vi "Arial Assist Ball Fetch.vi"() -> ()   [LabVIEW 2013]
uses:
  <vilib>/Rock Robotics/WPI/RobotDrive/WPI_RobotDriveMecanumDrive_Cartesian.vi
panel:
  in  "Vision?":bool
  in  "Far X":dbl
  in  "Far Less":dbl
  in  "Far Greater":dbl
  in  "Close Greater":dbl
  in  "Close Less":dbl
  in  "Close Threshold":dbl
  in  "Stopping Threshold":dbl
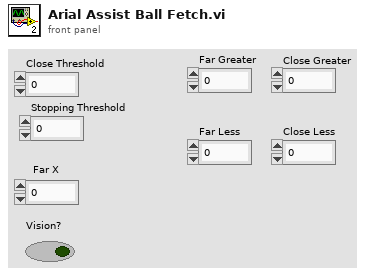
[diagram p1: front panel]
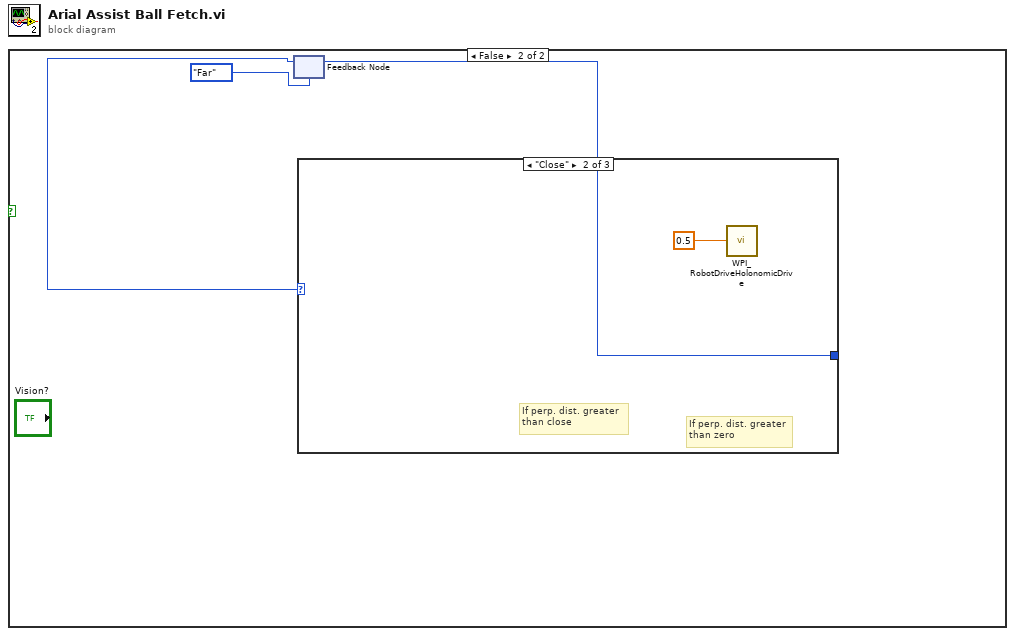
[diagram p0: block diagram]
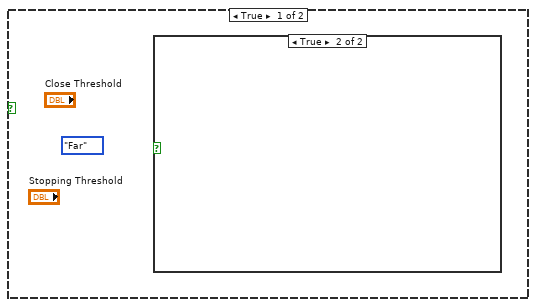
[diagram p2: hidden frame]
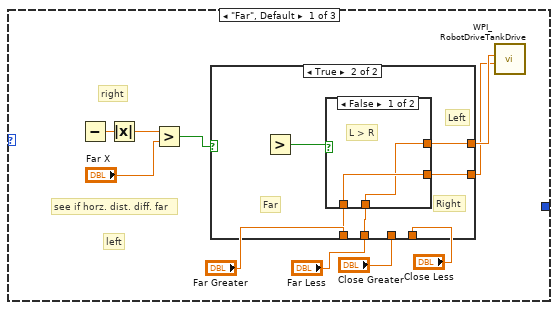
[diagram p4: hidden frame]
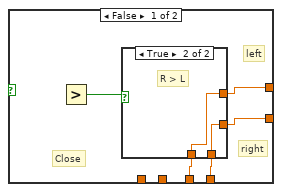
[diagram p5: hidden frame]
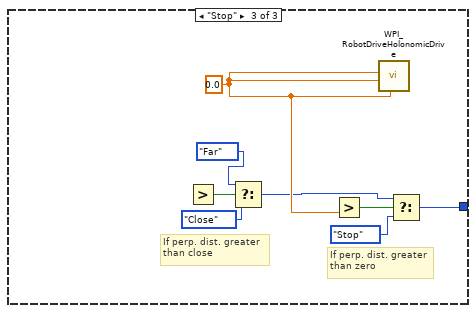
[diagram p8: hidden frame]
diagram:
  n1 = case shown="False" {
    selector: _ -> [_ _]
    frame True {
      (unwired) enum16{"Far", "Close", "Stop"}."Far"
      n2 = case shown="True" {
        selector: _ -> [_ _]
        frame False {
        }
        frame True {
        }
      }
    }
    frame False {
      n3 = feedback #1(enum16{"Far", "Close", "Stop"}."Far") -> (w2:enum16{"Far", "Close", "Stop"})
      n4 = case shown="\"Close\"" w2 {
        tunnel: [_ _ w33] -> w1
        frame "Far", Default {
          # "left"
          # "right"
          # "see if horz. dist. diff. far"
          n5 = Subtract() -> (x-y=w13:dbl)  [unwired: 2 in]
          n6 = Absolute Value(x=w13) -> (abs(x)=w12:dbl)
          n7 = Greater?(x=w12, y="Far X") -> (0:w10:bool)
          n8 = case shown="True" w10 {
            tunnel: [w17 w26] -> w9
            tunnel: [w16 w25] -> w8
            tunnel: "Close Less" -> [w15 _]
            tunnel: "Close Greater" -> [w14 _]
            tunnel: "Far Less" -> [_ w23]
            tunnel: "Far Greater" -> [_ w24]
            frame False {
              # "Close"
              # "right"
              # "left"
              n9 = Greater?() -> (0:w18:bool)  [unwired: 2 in]
              n10 = case shown="True" w18 {
                tunnel: [w19 w22] -> w17
                tunnel: [w20 w21] -> w16
                tunnel: w15 -> [w19 w21]
                tunnel: w14 -> [w20 w22]
                frame False {
                  # "L > R"
                }
                frame True {
                  # "R > L"
                }
              }
            }
            frame True {
              # "Right"
              # "Left"
              # "Far"
              n11 = Greater?() -> (0:w27:bool)  [unwired: 2 in]
              n12 = case shown="False" w27 {
                tunnel: [w28 w31] -> w26
                tunnel: [w29 w30] -> w25
                tunnel: w24 -> [w29 w31]
                tunnel: w23 -> [w28 w30]
                frame False {
                  # "L > R"
                }
                frame True {
                  # "R > L"
                }
              }
            }
          }
          n13 = call <vilib>:"WPI_RobotDriveTankDrive.vi"("Right axis value"=w8, "Left axis value"=w9) -> ()  [unwired: 7 in, 3 out]
        }
        frame "Close" {
          # "If perp. dist. greater\nthan zero"
          # "If perp. dist. greater \nthan close"
          n14 = call-poly <vilib>:"WPI_RobotDriveHolonomicDrive.vi"("Y"=0.5) -> ()  [unwired: 8 in, 3 out]
        }
        frame "Stop" {
          w36 = 0.0
          # "If perp. dist. greater\nthan zero"
          # "If perp. dist. greater \nthan close"
          n15 = Greater?() -> (0:w40:bool)  [unwired: 2 in]
          n16 = Select(t=enum16{"Far", "Close", "Stop"}."Far", s=w40, f=enum16{"Far", "Close", "Stop"}."Close") -> (s? t:f=w34:enum16{"Far", "Close", "Stop"})
          n17 = Greater?(y=w36) -> (0:w37:bool)  [unwired: 1 in]
          n18 = call-poly <vilib>:"WPI_RobotDriveHolonomicDrive.vi"("Rotation"=w36, "Y"=w36, "X"=w36) -> ()  [unwired: 6 in, 3 out]
          n19 = Select(t=w34, s=w37, f=enum16{"Far", "Close", "Stop"}."Stop") -> (s? t:f=w33:enum16{"Far", "Close", "Stop"})
        }
      }
      n20 = feedback-in #1(w1) -> ()
    }
  }
